vi "FITS_CreateImage.vi"(6 "bitpix code":i32=-32, 8 "error in":errorcluster, 9 "naxes":i64[](array[numeric]), 10 "naxis":i32, 11 "ref in":u64) -> (0 "error out":errorcluster, 3 "ref out":u64)   [LabVIEW 2016]
uses:
  usr/local/lib/libfits.so
panel:
  out "result":i32
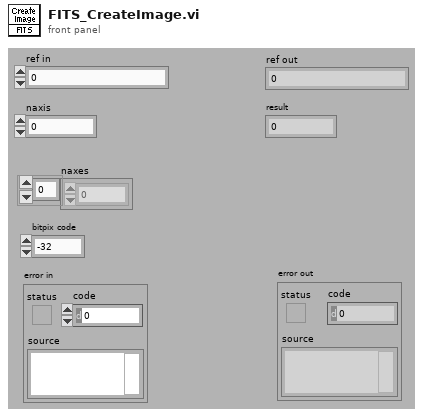
[diagram p1: front panel]
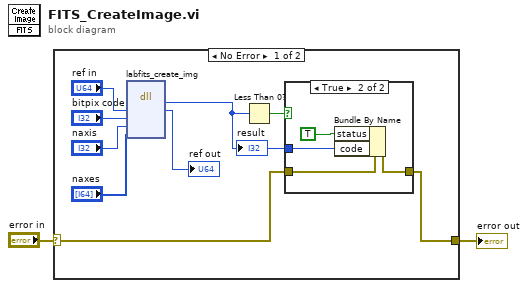
[diagram p0: block diagram]
diagram:
  n1 = case shown="No Error" "error in" {
    selector: "error in" -> [w10 w17]
    tunnel: [w9 w17] -> w1
    frame No Error {
      n2 = dll-call lib="usr/local/lib/libfits.so" fn="labfits_create_img" ("create image")("ref"="ref in", "bitpix"="bitpix code", "naxis"="naxis", "naxes"="naxes") -> ("return type"=w8:i32, "ref"=→"ref out":u64)  [unwired: 6 in, 2 out]
      "result" <- w8
      n3 = Less Than 0?(x=w8) -> (x < 0?=w11:bool)
      n4 = case shown="True" w11 {
        tunnel: w10 -> [w12 w14]
        tunnel: [w12 w13] -> w9
        tunnel: w8 -> [_ w15]
        frame False {
        }
        frame True {
          n5 = Bundle By Name(cluster=w14, "status"=TRUE, "code"=w15) -> (w13:errorcluster)
        }
      }
    }
    frame Error {
    }
  }
  "error out" <- w1
